vi "SeCrTs-RT_DAQ_Phase3.vi"(8 "error in":errorcluster, 11 "Data FIFO Ref":T1) -> (0 "error out":errorcluster)   [LabVIEW 2022 SP3]
uses:
  RT Controls/Data FIFO.ctl
  <vilib>/DAQmx/configure/timing.llb/DAQmx Timing (Sample Clock).vi
  <vilib>/DAQmx/configure/trigger.llb/DAQmx Start Trigger (Digital Edge).vi
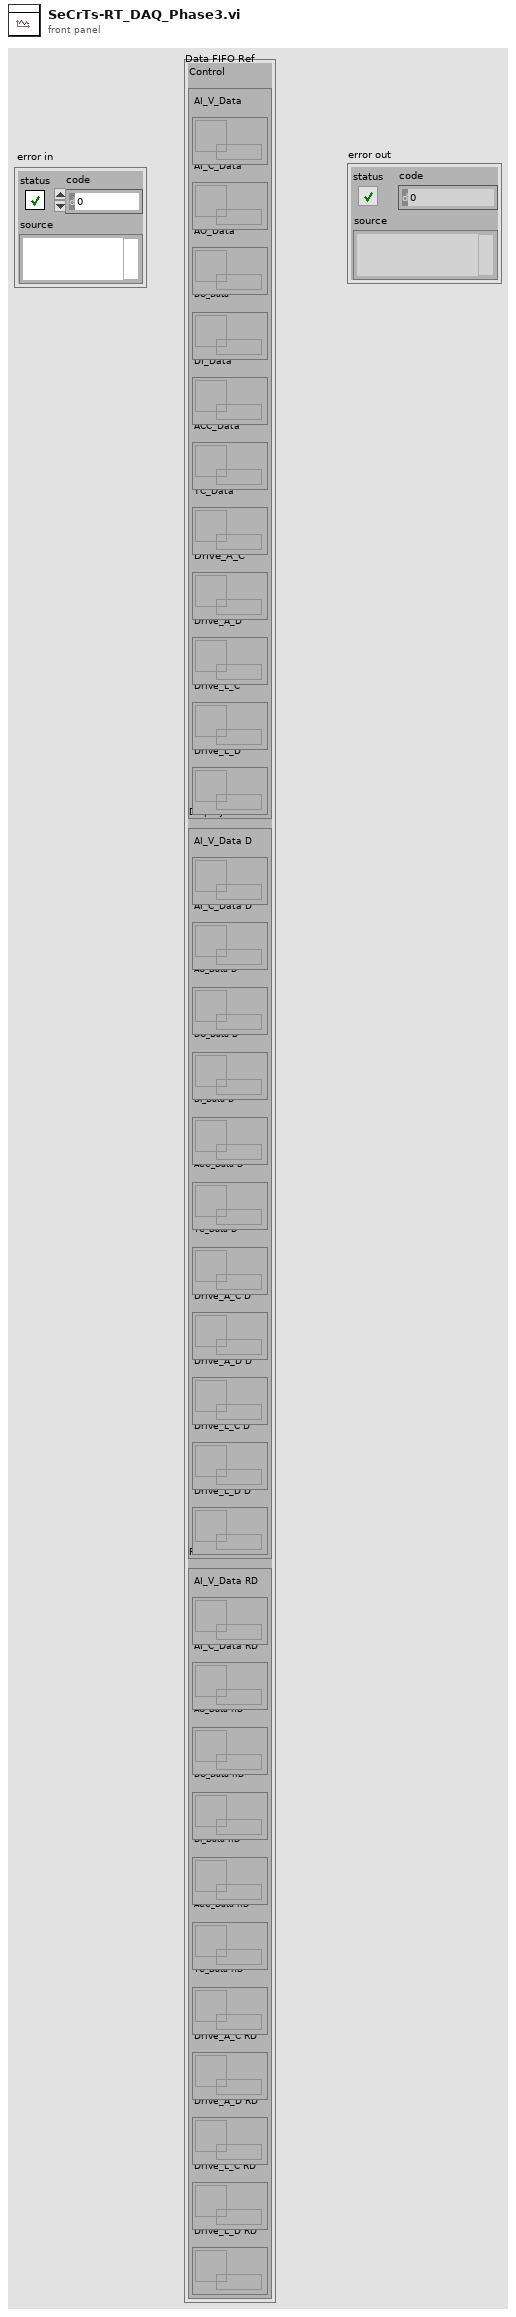
[diagram p1: front panel]
types:
  T1 = typedef "Data FIFO.ctl" = cluster{"Control":cluster{"AI_V_Data":refnum<queue>, "AI_C_Data":refnum<queue>, "AO_Data":refnum<queue>, "DO_Data":refnum<queue>, "DI_Data":refnum<queue>, "ACC_Data":refnum<queue>, "TC_Data":refnum<queue>, "Drive_A_C":refnum<queue>, "Drive_A_D":refnum<queue>, "Drive_L_C":refnum<queue>, "Drive_L_D":refnum<queue>}, "Display":cluster{"AI_V_Data D":refnum<queue>, "AI_C_Data D":refnum<queue>, "AO_Data D":refnum<queue>, "DO_Data D":refnum<queue>, "DI_Data D":refnum<queue>, "ACC_Data D":refnum<queue>, "TC_Data D":refnum<queue>, "Drive_A_C D":refnum<queue>, "Drive_A_D D":refnum<queue>, "Drive_L_C D":refnum<queue>, "Drive_L_D D":refnum<queue>}, "RD":cluster{"AI_V_Data RD":refnum<queue>, "AI_C_Data RD":refnum<queue>, "AO_Data RD":refnum<queue>, "DO_Data RD":refnum<queue>, "DI_Data RD":refnum<queue>, "ACC_Data RD":refnum<queue>, "TC_Data RD":refnum<queue>, "Drive_A_C RD":refnum<queue>, "Drive_A_D RD":refnum<queue>, "Drive_L_C RD":refnum<queue>, "Drive_L_D RD":refnum<queue>}}
  T2 = cluster{"AO config":cluster{"Channel_Name":string, "Channel_Number":string, "Default_Value":dbl, "Units":string}[], "AI config":cluster{"Channel_Name":string, "Channel_Number":string, "Pre_Scale_min":dbl, "Pre_Scale_max":dbl, "Sensor_min":dbl, "Sensor_max":dbl, "Units":string}[], "DI config":cluster{"Channel_Name":string, "Channel_Number":string, "Default_Value":bool, "DI invert?":bool}[], "DO config":cluster{"Channel_Name":string, "Channel_Number":string, "Default_Value":bool, "DO invert?":bool}[], "TC config":cluster{"Channel_Name":string, "Channel_Number":string, "Pre_Scale_min":dbl, "Pre_Scale_max":dbl, "units":i32, " type":i32}[], "ACC config":cluster{"Channel_Name":string, "Channel_Number":string, "Pre_Scale_min":dbl, "Pre_Scale_max":dbl, "Terminal configuration":i32, "Sensitivity":dbl, "Sensitivity units":i32}[], "SG config":cluster{"Channel_Name":string, "Channel_Number":string, "Pre_Scale_min":dbl, "Pre_Scale_max":dbl}[], "Strain Gauge Settings":cluster{"poisson ratio":dbl, "nominal gage resistance":dbl, "gage factor":dbl}, "Bridge Settings":cluster{"voltage excitation value":dbl, "voltage excitation source":i32, "initial bridge voltage":dbl, "lead wire resistance":dbl, "strain configuration":i32}, "Sample Rate":cluster{"AI Sample Rate":dbl[], "AO Sample Rate":dbl[], "DI Sample Rate":dbl[], "TC Sample Rate":dbl[], "DO Sample Rate":dbl[], "SG Sample Rate":dbl[], "ACC Sample Rate":dbl[]}}
  T3 = enum16{"Initialize", "Create Task", "Start", "Acquire", "Stop", "Exit"}
  T4 = cluster{"AI_Task":refnum<k21>, "AO_Task":refnum<k21>, "DI_Task":refnum<k21>, "DO_Task":refnum<k21>, "ACC_Task":refnum<k21>, "TC_Task":refnum<k21>, "AI_V_Task":refnum<k21>}
  T5 = cluster{"Start DAQ":bool, "Stop DAQ":bool, "RT Stop":bool, "RT Exit":bool}
  T6 = cluster{"AO config":cluster{"Channel_Name":string, "Channel_Number":string, "Default_Value":dbl, "Units":string}[], "AI config":cluster{"Channel_Name":string, "Channel_Number":string, "Pre_Scale_min":dbl, "Pre_Scale_max":dbl, "Sensor_min":dbl, "Sensor_max":dbl, "Units":string}[], "DI config":cluster{"Channel_Name":string, "Channel_Number":string, "Default_Value":bool, "DI invert?":bool}[], "DO config":cluster{"Channel_Name":string, "Channel_Number":string, "Default_Value":bool, "DO invert?":bool}[], "TC config":cluster{"Channel_Name":string, "Channel_Number":string, "Pre_Scale_min":dbl, "Pre_Scale_max":dbl, "units":i32, "thermocouple type":i32}[], "ACC config":cluster{"Channel_Name":string, "Channel_Number":string, "Pre_Scale_min":dbl, "Pre_Scale_max":dbl, "Terminal configuration":i32, "Sensitivity":dbl, "Sensitivity units":i32}[], "SG config":cluster{"Channel_Name":string, "Channel_Number":string, "Pre_Scale_min":dbl, "Pre_Scale_max":dbl}[], "Strain Gauge Settings":cluster{"poisson ratio":dbl, "nominal gage resistance":dbl, "gage factor":dbl}, "Bridge Settings":cluster{"voltage excitation value":dbl, "voltage excitation source":i32, "initial bridge voltage":dbl, "lead wire resistance":dbl, "strain configuration":i32}, "Sample Rate":cluster{"AI Sample Rate":dbl[], "AO Sample Rate":dbl[], "DI Sample Rate":dbl[], "TC Sample Rate":dbl[], "DO Sample Rate":dbl[], "SG Sample Rate":dbl[], "ACC Sample Rate":dbl[]}}
  T7 = cluster{"Channel_Name":string, "Channel_Number":string, "Pre_Scale_min":dbl, "Pre_Scale_max":dbl, "Sensor_min":dbl, "Sensor_max":dbl, "Units":string}[]
  T8 = cluster{"Channel_Name":string, "Channel_Number":string, "Default_Value":dbl, "Units":string}[]
  T9 = cluster{"Channel_Name":string, "Channel_Number":string, "Default_Value":bool, "DI invert?":bool}[]
  T10 = cluster{"Channel_Name":string, "Channel_Number":string, "Default_Value":bool, "DO invert?":bool}[]
  T11 = cluster{"Channel_Name":string, "Channel_Number":string, "Pre_Scale_min":dbl, "Pre_Scale_max":dbl, "Terminal configuration":i32, "Sensitivity":dbl, "Sensitivity units":i32}[]
  T12 = cluster{"Channel_Name":string, "Channel_Number":string, "Pre_Scale_min":dbl, "Pre_Scale_max":dbl, "units":i32, " type":i32}[]
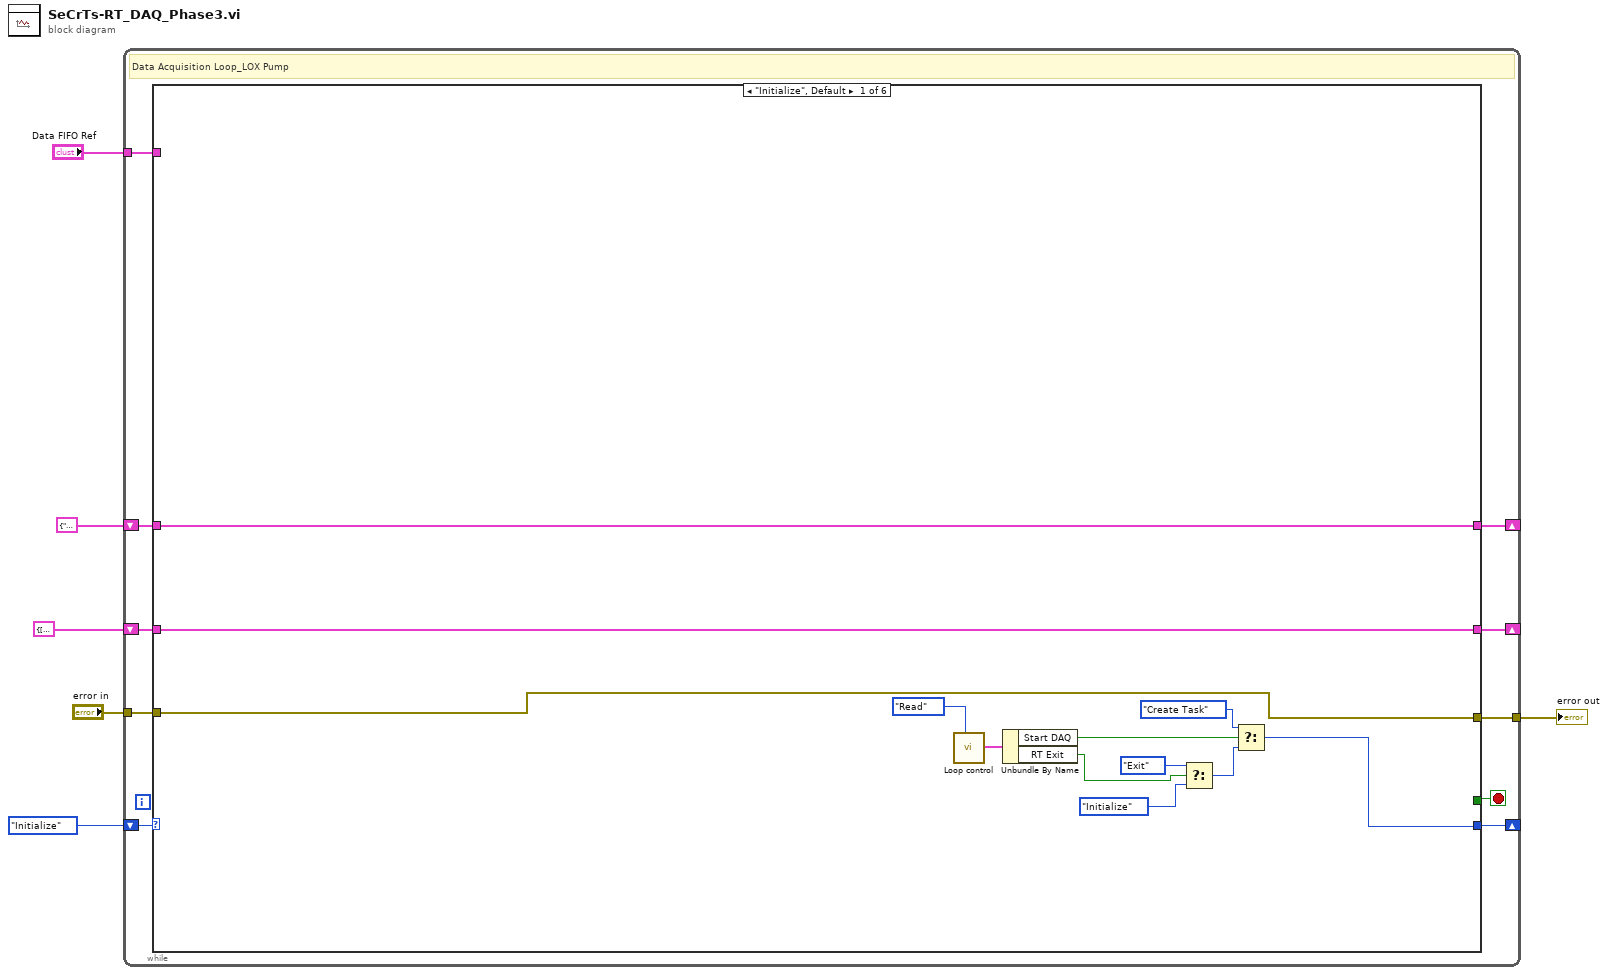
[diagram p0: block diagram]
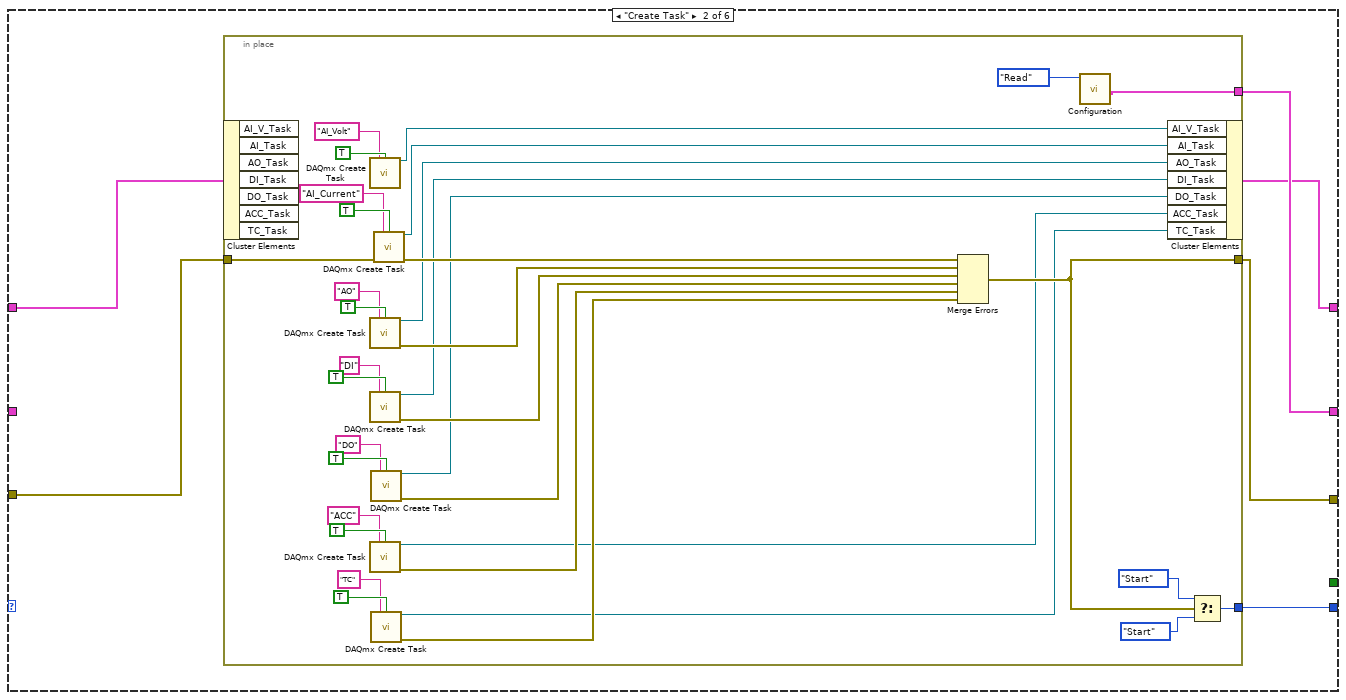
[diagram p2: hidden frame]
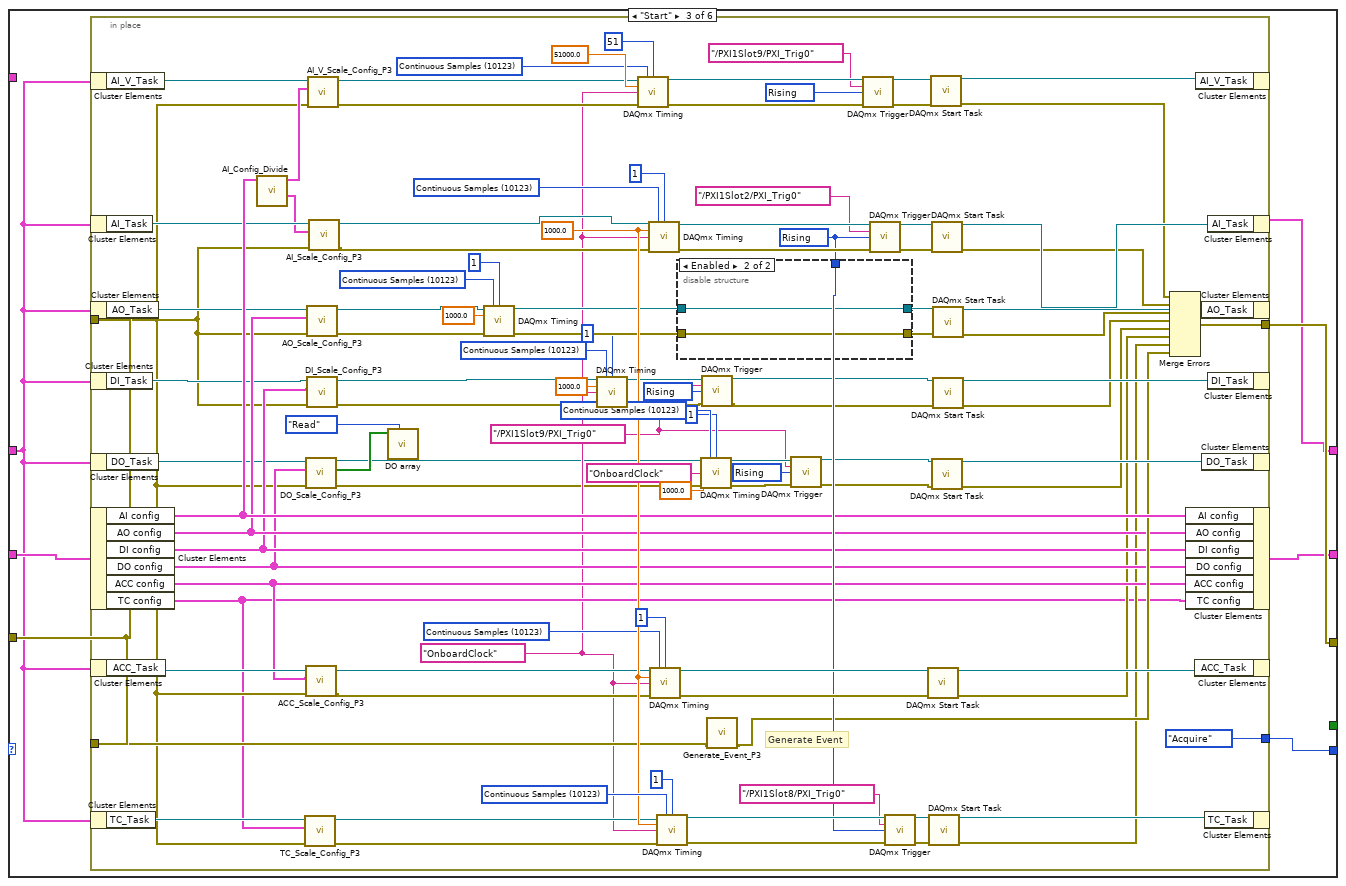
[diagram p3: hidden frame]
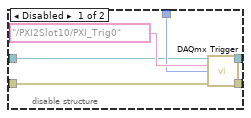
[diagram p4: hidden frame]
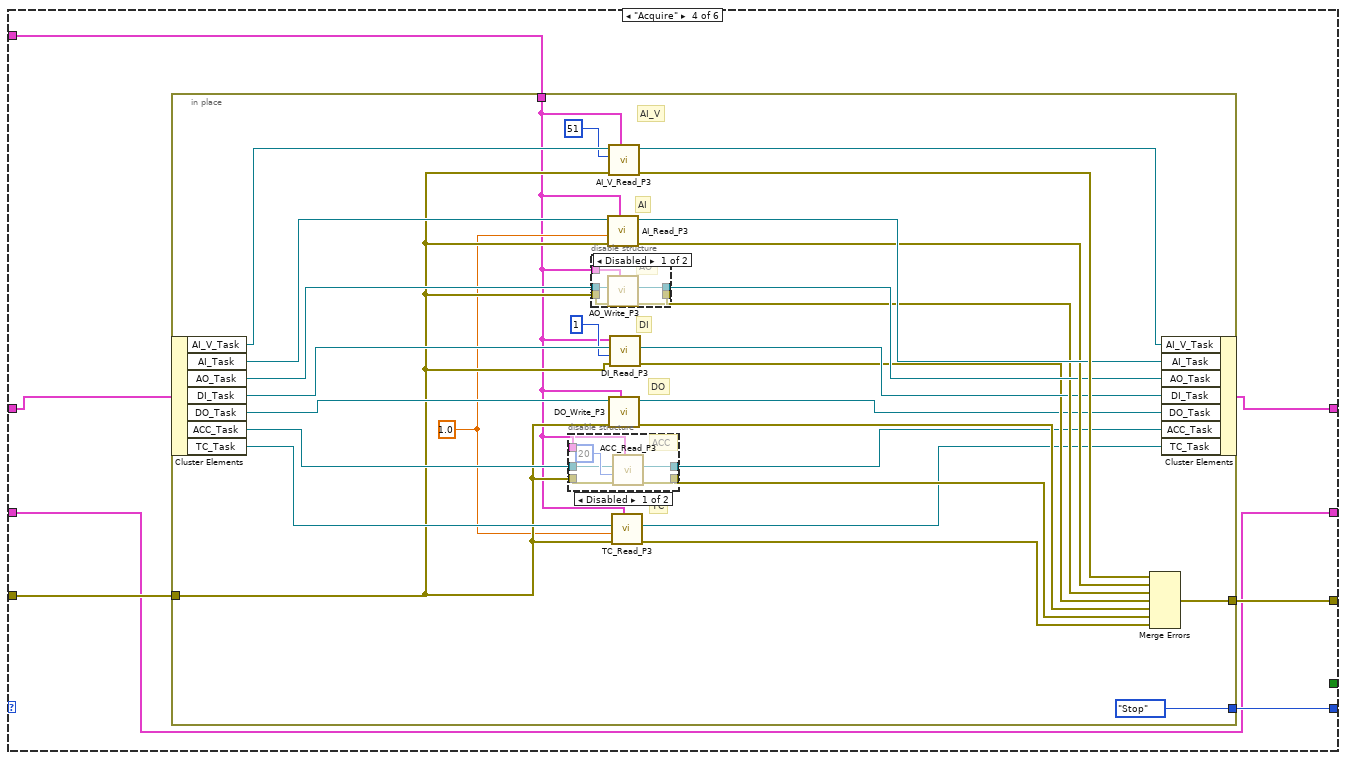
[diagram p5: hidden frame]
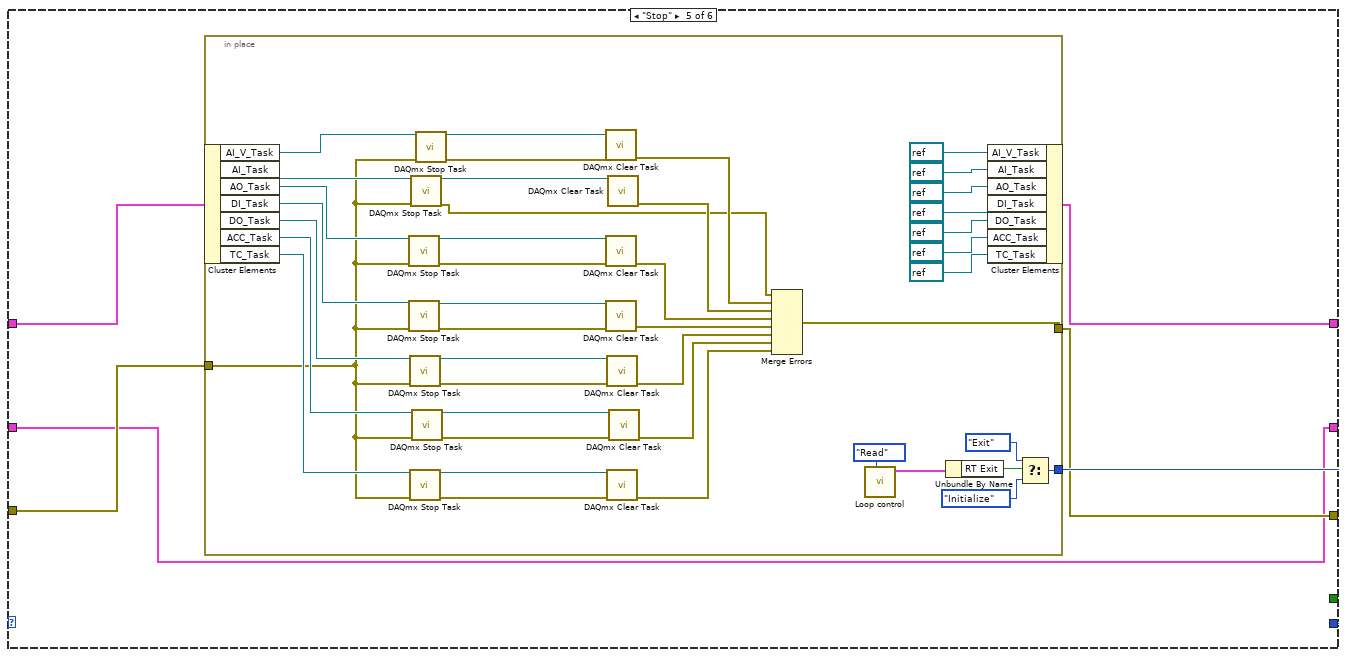
[diagram p8: hidden frame]
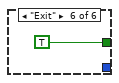
[diagram p9: hidden frame]
diagram:
  n1 = while {
    shift-right: [w13] -> _
    shift-left: T3."Initialize" -> [w16]
    tunnel: "error in" -> [w15]
    tunnel: [w14] -> w5
    shift-right: [w10] -> _
    shift-left: T2 {"AO config"=[], "AI config"=[], "DI config"=[], "DO config"=[], "TC config"=[], "ACC config"=[], "SG config"=[], "Strain Gauge Settings"={"poisson ratio"=0.0, "nominal gage resistance"=0.0, "gage factor"=0.0}, "Bridge Settings"={"voltage excitation value"=0.0, "voltage excitation source"=0, "initial bridge voltage"=0.0, "lead wire resistance"=0.0, "strain configuration"=0}, "Sample Rate"={"AI Sample Rate"=[], "AO Sample Rate"=[], "DI Sample Rate"=[], "TC Sample Rate"=[], "DO Sample Rate"=[], "SG Sample Rate"=[], "ACC Sample Rate"=[]}} ("Config out") -> [w11]
    shift-right: [w8] -> _
    shift-left: T4 {"AI_Task"="", "AO_Task"="", "DI_Task"="", "DO_Task"="", "ACC_Task"="", "TC_Task"="", "AI_V_Task"=""} -> [w12]
    tunnel: "Data FIFO Ref" -> [w7]
    stop <- w9 stop-if-true
    # "Data Acquisition Loop_LOX Pump"
    n2 = case shown="\"Initialize\", Default" w16 {
      tunnel: w15 -> [w23 w33 w70 w194 w238 _]
      tunnel: [w23 w32 w74 w193 w239 _] -> w14
      tunnel: [w27 w31 w75 w195 w240 _] -> w13
      tunnel: w12 -> [w18 w30 w69 w192 w237 _]
      tunnel: w11 -> [w17 _ w72 w190 w235 _]
      tunnel: [w17 w34 w73 w190 w235 _] -> w10
      tunnel: [_ _ _ _ _ TRUE] -> w9
      tunnel: [w18 w29 w71 w191 w236 _] -> w8
      tunnel: w7 -> [_ _ _ w189 _ _]
      frame "Initialize", Default {
        n3 = call "Loop control.vi"("Action"=enum16{"Init", "Write", "Read"}."Read") -> ("Loop Control Out"=w22:T5)  [unwired: 9 in, 1 out]
        n4 = Unbundle By Name(w22) -> ("Start DAQ"=w21:bool, "RT Exit"=w20:bool)
        n5 = Select(t=T3."Exit", s=w20, f=T3."Initialize") -> (s? t:f=w24:T3)
        n6 = Select(t=T3."Create Task", s=w21, f=w24) -> (s? t:f=w27:T3)
      }
      frame "Create Task" {
        n7 = in-place "In Place Element Structure" {
          in-place-border: [w43] -> w34
          in-place-border: w33 -> [w47]
          in-place-border: [w56] -> w32
          in-place-border: [w54] -> w31
          n8 = in-place-cluster #1(w30) -> ()  [unwired: 7 out]
          n9 = call <vilib>:"DAQmx Create Task.vi"("new task name"="AI_Volt", "auto cleanup"=TRUE) -> ("task out"=w44:refnum<k21>)  [unwired: 12 in, 1 out]
          n10 = call <vilib>:"DAQmx Create Task.vi"("new task name"="AO", "auto cleanup"=TRUE) -> ("task out"=w52:refnum<k21>, "error out"=w62:errorcluster)  [unwired: 12 in]
          n11 = call <vilib>:"DAQmx Create Task.vi"("new task name"="DI", "auto cleanup"=TRUE) -> ("task out"=w51:refnum<k21>, "error out"=w61:errorcluster)  [unwired: 12 in]
          n12 = call <vilib>:"DAQmx Create Task.vi"("new task name"="ACC", "auto cleanup"=TRUE) -> ("task out"=w49:refnum<k21>, "error out"=w59:errorcluster)  [unwired: 12 in]
          n13 = call <vilib>:"DAQmx Create Task.vi"("new task name"="DO", "auto cleanup"=TRUE) -> ("task out"=w50:refnum<k21>, "error out"=w60:errorcluster)  [unwired: 12 in]
          n14 = call <vilib>:"DAQmx Create Task.vi"("new task name"="TC", "auto cleanup"=TRUE) -> ("task out"=w48:refnum<k21>, "error out"=w58:errorcluster)  [unwired: 12 in]
          n15 = call <vilib>:"DAQmx Create Task.vi"("new task name"="AI_Current", "auto cleanup"=TRUE, "error in"=w47) -> ("task out"=w53:refnum<k21>, "error out"=w68:errorcluster)  [unwired: 11 in]
          n16 = Merge Errors(w68, w62, w61, w60, w59, w58) -> (w56:errorcluster)
          n17 = call "Configuration.vi"("Enum"=enum16{"Write", "Read"}."Read") -> ("Config out"=w43:T6)  [unwired: 10 in]
          n18 = in-place-cluster #1("AI_V_Task"=w44, "AI_Task"=w53, "AO_Task"=w52, "DI_Task"=w51, "DO_Task"=w50, "ACC_Task"=w49, "TC_Task"=w48) -> (w29:T4)
          n19 = Select(t=T3."Start", s=w56, f=T3."Start") -> (s? t:f=w54:T3)
        }
      }
      frame "Start" {
        n20 = in-place "In Place Element Structure" {
          in-place-border: [T3."Acquire"] -> w75
          in-place-border: [w178] -> w74
          in-place-border: w70 -> [w114]
          in-place-border: w70 -> [w133]
          w76 = 10280 items=["Rising"=10280, "Falling"=10171] ("edge")
          w83 = 10123 items=["Finite Samples"=10178, "Continuous Samples"=10123, "Hardware Timed Single Point"=12522] ("sample mode")
          w91 = 10280 items=["Rising"=10280, "Falling"=10171] ("edge")
          w77 = tag "/PXI1Slot9/PXI_Trig0" ("source")
          w96 = 10123 items=["Finite Samples"=10178, "Continuous Samples"=10123, "Hardware Timed Single Point"=12522] ("sample mode")
          w99 = 10123 items=["Finite Samples"=10178, "Continuous Samples"=10123, "Hardware Timed Single Point"=12522] ("sample mode")
          w97 = tag "OnboardClock" ("source")
          w103 = 10280 items=["Rising"=10280, "Falling"=10171] ("edge")
          w146 = 10123 items=["Finite Samples"=10178, "Continuous Samples"=10123, "Hardware Timed Single Point"=12522] ("sample mode")
          w150 = 10123 items=["Finite Samples"=10178, "Continuous Samples"=10123, "Hardware Timed Single Point"=12522] ("sample mode")
          w155 = 10280 items=["Rising"=10280, "Falling"=10171] ("edge")
          w167 = 1000.0 ("number")
          w177 = 10123 items=["Finite Samples"=10178, "Continuous Samples"=10123, "Hardware Timed Single Point"=12522] ("sample mode")
          w176 = 10123 items=["Finite Samples"=10178, "Continuous Samples"=10123, "Hardware Timed Single Point"=12522] ("sample mode")
          # "Generate Event"
          n21 = in-place-cluster #2(w69) -> ("AI_V_Task"=w136:refnum<k21>)
          n22 = in-place-cluster #3(w69) -> ("AI_Task"=w130:refnum<k21>)
          n23 = in-place-cluster #4(w69) -> ("AO_Task"=w127:refnum<k21>)
          n24 = in-place-cluster #5(w69) -> ("DI_Task"=w125:refnum<k21>)
          n25 = in-place-cluster #6(w69) -> ("DO_Task"=w123:refnum<k21>)
          n26 = in-place-cluster #7(w72) -> ("AI config"=w149:T7, "AO config"=w126:T8, "DI config"=w124:T9, "DO config"=w121:T10, "ACC config"=w117:T11, "TC config"=w104:T12)
          n27 = in-place-cluster #8(w69) -> ("ACC_Task"=w118:refnum<k21>)
          n28 = in-place-cluster #9(w69) -> ("TC_Task"=w116:refnum<k21>)
          n29 = call "AI_Config_Divide.vi"("AI config"=w149) -> ("AI C"=w112:T7, "AI V"=w135:T7)  [unwired: 9 in]
          n30 = call "TC_Scale_Config_P3.vi"("error in (no error)"=w114, "TC config"=w104, "Refnum in"=w116) -> ("error out"=w113:errorcluster, "Refnum out"=w115:refnum<k21>)  [unwired: 7 in]
          n31 = call "DO_Scale_Config_P3.vi"("error in (no error)"=w114, "DO config"=w121, "Refnum in"=w123) -> ("error out"=w87:errorcluster, "Array"=w122:bool[], "Refnum out"=w86:refnum<k21>)  [unwired: 6 in]
          n32 = call "ACC_Scale_Config_P3.vi"("error in (no error)"=w114, "ACC config"=w117, "Refnum in"=w118) -> ("error out"=w120:errorcluster, "Refnum out"=w119:refnum<k21>)  [unwired: 7 in]
          n33 = call "AO_Scale_Config_P3.vi"("error in (no error)"=w114, "AO config"=w126, "Refnum in"=w127) -> ("error out"=w129:errorcluster, "Refnum out"=w128:refnum<k21>)  [unwired: 7 in]
          n34 = call "DI_Scale_Config_P3.vi"("error in (no error)"=w114, "DI config"=w124, "Refnum in"=w125) -> ("error out"=w101:errorcluster, "Refnum out"=w100:refnum<k21>)  [unwired: 7 in]
          n35 = call "AI_V_Scale_Config_P3.vi"("error in"=w114, "AI C"=w135, "task in"=w136) -> ("error out"=w138:errorcluster, "task out"=w137:refnum<k21>)  [unwired: 7 in]
          n36 = call "AI_Scale_Config_P3.vi"("error in (no error)"=w114, "AI C"=w112, "Refnum in"=w130) -> ("error out"=w131:errorcluster, "Refnum out"=w132:refnum<k21>)  [unwired: 7 in]
          n37 = call "DO array.vi"("Enum"=enum16{"Write", "Read"}."Read", "DO Array"=w122) -> ()  [unwired: 10 in]
          n38 = call-poly <vilib>:"DAQmx Timing.vi"("task/channels in"=w128, "sample mode"=w150, "samples per channel"=1, "rate"=1000.0, "error in"=w129) -> ("task out"=w154:refnum<k21>, "error out"=w153:errorcluster)  [unwired: 9 in]
          n39 = call-poly <vilib>:"DAQmx Timing.vi"("task/channels in"=w100, "sample mode"=w96, "samples per channel"=1, "rate"=1000.0, "source"=w97, "error in"=w101) -> ("task out"=w93:refnum<k21>, "error out"=w92:errorcluster)  [unwired: 8 in]
          n40 = call-poly <vilib>:"DAQmx Timing.vi"("task/channels in"=w137, "sample mode"=w146, "samples per channel"=51, "rate"=51000.0 ("samples per channel"), "source"=w97, "error in"=w138) -> ("task out"=w144:refnum<k21>, "error out"=w145:errorcluster)  [unwired: 8 in]
          n41 = call-poly <vilib>:"DAQmx Timing.vi"("task/channels in"=w132, "sample mode"=w176, "samples per channel"=1, "rate"=w167, "source"=w97, "error in"=w131) -> ("task out"=w180:refnum<k21>, "error out"=w165:errorcluster)  [unwired: 8 in]
          n42 = call-poly <vilib>:"DAQmx Timing.vi"("task/channels in"=w119, "sample mode"=w99, "samples per channel"=1, "rate"=w167, "source"=w97, "error in"=w120) -> ("task out"=w161:refnum<k21>, "error out"=w160:errorcluster)  [unwired: 8 in]
          n43 = call-poly <vilib>:"DAQmx Timing.vi"("task/channels in"=w115, "sample mode"=w177, "samples per channel"=1, "rate"=w167, "source"=w97, "error in"=w113) -> ("task out"=w159:refnum<k21>, "error out"=w156:errorcluster)  [unwired: 8 in]
          n44 = disable-structure shown="Enabled" {
            disable-tunnel: [w186 w188] -> w163
            disable-tunnel: [w185 w187] -> w162
            disable-tunnel: w155 -> [w183 _]
            disable-tunnel: w154 -> [w182 w188]
            disable-tunnel: w153 -> [w181 w187]
            frame Disabled {
              n45 = call-poly <vilib>:"DAQmx Trigger.vi"("task/channels in"=w182, "source"=tag "/PXI2Slot10/PXI_Trig0", "edge"=w183, "error in"=w181) -> ("task out"=w186:refnum<k21>, "error out"=w185:errorcluster)  [unwired: 10 in]
            }
            frame Enabled {
            }
          }
          n46 = call-poly <vilib>:"DAQmx Timing.vi"("task/channels in"=w86, "sample mode"=w83, "samples per channel"=1, "rate"=1000.0, "source"=tag "OnboardClock", "error in"=w87) -> ("task out"=w80:refnum<k21>, "error out"=w81:errorcluster)  [unwired: 8 in]
          n47 = call-poly <vilib>:"DAQmx Trigger.vi"("task/channels in"=w93, "source"=w77, "edge"=w91, "error in"=w92) -> ("task out"=w90:refnum<k21>, "error out"=w89:errorcluster)  [unwired: 10 in]
          n48 = call "Generate_Event_P3.vi"("error in"=w133) -> ("error out"=w134:errorcluster)  [unwired: 10 in]
          n49 = call-poly <vilib>:"DAQmx Trigger.vi"("task/channels in"=w80, "source"=w77, "edge"=w76, "error in"=w81) -> ("task out"=w79:refnum<k21>, "error out"=w78:errorcluster)  [unwired: 10 in]
          n50 = call-poly <vilib>:"DAQmx Trigger.vi"("task/channels in"=w144, "source"=tag "/PXI1Slot9/PXI_Trig0", "edge"=w103, "error in"=w145) -> ("task out"=w141:refnum<k21>, "error out"=w142:errorcluster)  [unwired: 10 in]
          n51 = call-poly <vilib>:"DAQmx Trigger.vi"("task/channels in"=w180, "source"=tag "/PXI1Slot2/PXI_Trig0", "edge"=w155, "error in"=w165) -> ("task out"=w166:refnum<k21>, "error out"=w164:errorcluster)  [unwired: 10 in]
          n52 = call-poly <vilib>:"DAQmx Trigger.vi"("task/channels in"=w159, "source"=tag "/PXI1Slot8/PXI_Trig0", "edge"=w155, "error in"=w156) -> ("task out"=w158:refnum<k21>, "error out"=w157:errorcluster)  [unwired: 10 in]
          n53 = call <vilib>:"DAQmx Start Task.vi"("task/channels in"=w161, "error in"=w160) -> ("task out"=w170:refnum<k21>, "error out"=w106:errorcluster)  [unwired: 12 in]
          n54 = call <vilib>:"DAQmx Start Task.vi"("task/channels in"=w158, "error in"=w157) -> ("task out"=w171:refnum<k21>, "error out"=w105:errorcluster)  [unwired: 12 in]
          n55 = call <vilib>:"DAQmx Start Task.vi"("task/channels in"=w141, "error in"=w142) -> ("task out"=w140:refnum<k21>, "error out"=w111:errorcluster)  [unwired: 12 in]
          n56 = call <vilib>:"DAQmx Start Task.vi"("task/channels in"=w166, "error in"=w164) -> ("task out"=w173:refnum<k21>, "error out"=w110:errorcluster)  [unwired: 12 in]
          n57 = call <vilib>:"DAQmx Start Task.vi"("task/channels in"=w79, "error in"=w78) -> ("task out"=w169:refnum<k21>, "error out"=w107:errorcluster)  [unwired: 12 in]
          n58 = call <vilib>:"DAQmx Start Task.vi"("task/channels in"=w163, "error in"=w162) -> ("task out"=w172:refnum<k21>, "error out"=w109:errorcluster)  [unwired: 12 in]
          n59 = call <vilib>:"DAQmx Start Task.vi"("task/channels in"=w90, "error in"=w89) -> ("task out"=w168:refnum<k21>, "error out"=w108:errorcluster)  [unwired: 12 in]
          n60 = Merge Errors(w111, w110, w109, w108, w107, w106, w105, w134) -> (w178:errorcluster)
          n61 = in-place-cluster #7("AI config"=w149, "AO config"=w126, "DI config"=w124, "DO config"=w121, "ACC config"=w117, "TC config"=w104) -> (w73:T2)
          n62 = in-place-cluster #8("ACC_Task"=w170) -> ()  [unwired: 1 out]
          n63 = in-place-cluster #2("AI_V_Task"=w140) -> ()  [unwired: 1 out]
          n64 = in-place-cluster #4("AO_Task"=w172) -> ()  [unwired: 1 out]
          n65 = in-place-cluster #6("DO_Task"=w169) -> ()  [unwired: 1 out]
          n66 = in-place-cluster #9("TC_Task"=w171) -> ()  [unwired: 1 out]
          n67 = in-place-cluster #3("AI_Task"=w173) -> (w71:T4)
          n68 = in-place-cluster #5("DI_Task"=w168) -> ()  [unwired: 1 out]
        }
      }
      frame "Acquire" {
        n69 = in-place "In Place Element Structure" {
          in-place-border: [T3."Stop"] -> w195
          in-place-border: w194 -> [w200]
          in-place-border: [w222] -> w193
          in-place-border: w189 -> [w196]
          w199 = 1.0
          # "AI_V"
          # "TC"
          # "DO"
          # "DI"
          # "AI"
          n70 = in-place-cluster #10(w192) -> ("AI_V_Task"=w219:refnum<k21>, "AI_Task"=w218:refnum<k21>, "AO_Task"=w214:refnum<k21>, "DI_Task"=w211:refnum<k21>, "DO_Task"=w208:refnum<k21>, "ACC_Task"=w205:refnum<k21>, "TC_Task"=w203:refnum<k21>)
          n71 = disable-structure shown="Disabled" {
            disable-tunnel: [w228 _] -> w206
            disable-tunnel: w205 -> [w227 _]
            disable-tunnel: [w226 _] -> w204
            disable-tunnel: w200 -> [w225 _]
            disable-tunnel: w196 -> [w224 _]
            frame Disabled {
              # "ACC"
              n72 = call "ACC_Read_P3.vi"("Data FIFO Ref"=w224, "error in (no error)"=w225, "number of samples per channel"=20, "ACC_Task"=w227) -> ("error out"=w226:errorcluster, "task out"=w228:refnum<k21>)  [unwired: 6 in]
            }
            frame Enabled {
            }
          }
          n73 = disable-structure shown="Disabled" {
            disable-tunnel: [w234 _] -> w215
            disable-tunnel: w214 -> [w233 _]
            disable-tunnel: [w232 _] -> w213
            disable-tunnel: w200 -> [w231 _]
            disable-tunnel: w196 -> [w230 _]
            frame Disabled {
              # "AO"
              n74 = call "AO_Write_P3.vi"("Data FIFO Ref"=w230, "error in (no error)"=w231, "AO_Task"=w233) -> ("error out"=w232:errorcluster, "task out"=w234:refnum<k21>)  [unwired: 7 in]
            }
            frame Enabled {
            }
          }
          n75 = call "AI_Read_P3.vi"("Data FIFO Ref"=w196, "error in (no error)"=w200, "Numeric"=w199, "AI_Task"=w218) -> ("error out"=w216:errorcluster, "task out"=w217:refnum<k21>)  [unwired: 4 in]
          n76 = call "AI_V_Read_P3.vi"("Data FIFO Ref"=w196, "error in"=w200, "number of samples per channel"=51, "AI_V_Task"=w219) -> ("error out"=w221:errorcluster, "AI_V_Task"=w220:refnum<k21>)  [unwired: 6 in]
          n77 = call "DO_Write_P3.vi"("Data FIFO Ref"=w196, "error in (no error)"=w200, "Refnum in"=w208) -> ("error out"=w207:errorcluster, "Refnum out"=w209:refnum<k21>)  [unwired: 7 in]
          n78 = call "DI_Read_P3.vi"("error in (no error)"=w200, "number of samples per channel"=1, "DI_Task"=w211, "Data FIFO Ref"=w196) -> ("error out"=w210:errorcluster, "task out"=w212:refnum<k21>)  [unwired: 6 in]
          n79 = call "TC_Read_P3.vi"("Data FIFO Ref"=w196, "error in (no error)"=w200, "Numeric"=w199, "TC_Task"=w203) -> ("error out"=w201:errorcluster, "task out"=w202:refnum<k21>)  [unwired: 6 in]
          n80 = Merge Errors(w221, w216, w213, w210, w207, w204, w201) -> (w222:errorcluster)
          n81 = in-place-cluster #10("AI_V_Task"=w220, "AI_Task"=w217, "AO_Task"=w215, "DI_Task"=w212, "DO_Task"=w209, "ACC_Task"=w206, "TC_Task"=w202) -> (w191:T4)
        }
      }
      frame "Stop" {
        n82 = in-place "In Place Element Structure" {
          in-place-border: [w280] -> w240
          in-place-border: [w274] -> w239
          in-place-border: w238 -> [w255]
          n83 = in-place-cluster #11(w237) -> ("AI_V_Task"=w257:refnum<k21>, "AI_Task"=w266:refnum<k21>, "AO_Task"=w265:refnum<k21>, "DI_Task"=w268:refnum<k21>, "DO_Task"=w267:refnum<k21>, "ACC_Task"=w264:refnum<k21>, "TC_Task"=w263:refnum<k21>)
          n84 = call <vilib>:"DAQmx Stop Task.vi"("task/channels in"=w265, "error in"=w255) -> ("task out"=w262:refnum<k21>, "error out"=w279:errorcluster)  [unwired: 12 in]
          n85 = call <vilib>:"DAQmx Stop Task.vi"("task/channels in"=w268, "error in"=w255) -> ("task out"=w261:refnum<k21>, "error out"=w278:errorcluster)  [unwired: 12 in]
          n86 = call <vilib>:"DAQmx Stop Task.vi"("task/channels in"=w267, "error in"=w255) -> ("task out"=w260:refnum<k21>, "error out"=w277:errorcluster)  [unwired: 12 in]
          n87 = call <vilib>:"DAQmx Stop Task.vi"("task/channels in"=w263, "error in"=w255) -> ("task out"=w258:refnum<k21>, "error out"=w275:errorcluster)  [unwired: 12 in]
          n88 = call <vilib>:"DAQmx Stop Task.vi"("task/channels in"=w266, "error in"=w255) -> ("task out"=w241:refnum<k21>, "error out"=w242:errorcluster)  [unwired: 12 in]
          n89 = call <vilib>:"DAQmx Stop Task.vi"("task/channels in"=w264, "error in"=w255) -> ("task out"=w259:refnum<k21>, "error out"=w276:errorcluster)  [unwired: 12 in]
          n90 = call <vilib>:"DAQmx Stop Task.vi"("task/channels in"=w257, "error in"=w255) -> ("task out"=w256:refnum<k21>, "error out"=w254:errorcluster)  [unwired: 12 in]
          n91 = call <vilib>:"DAQmx Clear Task.vi"("task in"=w256, "error in"=w254) -> ("error out"=w253:errorcluster)  [unwired: 13 in]
          n92 = call <vilib>:"DAQmx Clear Task.vi"("task in"=w262, "error in"=w279) -> ("error out"=w273:errorcluster)  [unwired: 13 in]
          n93 = call <vilib>:"DAQmx Clear Task.vi"("task in"=w261, "error in"=w278) -> ("error out"=w272:errorcluster)  [unwired: 13 in]
          n94 = call <vilib>:"DAQmx Clear Task.vi"("task in"=w260, "error in"=w277) -> ("error out"=w271:errorcluster)  [unwired: 13 in]
          n95 = call <vilib>:"DAQmx Clear Task.vi"("task in"=w258, "error in"=w275) -> ("error out"=w269:errorcluster)  [unwired: 13 in]
          n96 = call <vilib>:"DAQmx Clear Task.vi"("task in"=w241) -> ("error out"=w283:errorcluster)  [unwired: 14 in]
          n97 = call <vilib>:"DAQmx Clear Task.vi"("task in"=w259, "error in"=w276) -> ("error out"=w270:errorcluster)  [unwired: 13 in]
          n98 = Merge Errors(w242, w253, w283, w273, w272, w271, w270, w269) -> (w274:errorcluster)
          n99 = call "Loop control.vi"("Action"=enum16{"Init", "Write", "Read"}."Read") -> ("Loop Control Out"=w252:T5)  [unwired: 9 in, 1 out]
          n100 = Unbundle By Name(w252) -> ("RT Exit"=w251:bool)
          n101 = in-place-cluster #11("AI_V_Task"=refnum<k21> refnum, "AI_Task"=refnum<k21> refnum, "AO_Task"=refnum<k21> refnum, "DI_Task"=refnum<k21> refnum, "DO_Task"=refnum<k21> refnum, "ACC_Task"=refnum<k21> refnum, "TC_Task"=refnum<k21> refnum) -> (w236:T4)
          n102 = Select(t=T3."Exit", s=w251, f=T3."Initialize") -> (s? t:f=w280:T3)
        }
      }
      frame "Exit" {
      }
    }
  }
  "error out" <- w5
